vi "Start.vi"(8 "error in (no error)":errorcluster, 11 "Execution Unit Implementation in":refnum<class "Execution Unit Implementation.lvclass">) -> (0 "error out":errorcluster, 3 "Execution Unit Implementation out":refnum<class "Execution Unit Implementation.lvclass">)   [LabVIEW 2020, in "Protocol Implementation.lvlib" / "Execution Unit Implementation.lvclass"]
uses:
  Execution Unit Implementation.lvclass
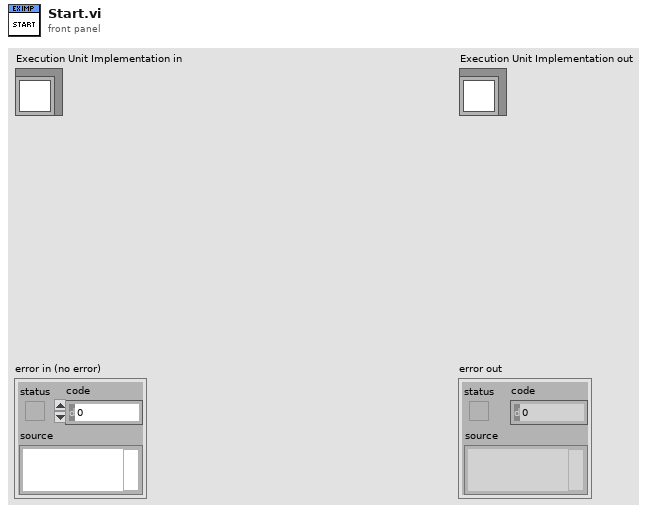
[diagram p1: front panel]
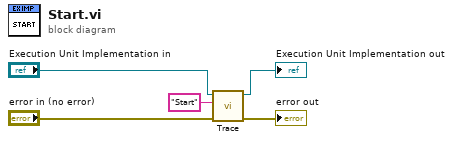
[diagram p0: block diagram]
diagram:
  n1 = call "Trace.vi"("Execution Unit Implementation in"="Execution Unit Implementation in", "message"="Start", "error in (no error)"="error in (no error)") -> ("Execution Unit Implementation out"=→"Execution Unit Implementation out":refnum<class "Execution Unit Implementation.lvclass">, "error out"=→"error out":errorcluster)  [unwired: 6 in]
